vi "Read GObjects.vi"(8 "error in (no error)":errorcluster, 11 "LangData in":refnum<class "VI Data.lvclass">) -> (0 "error out":errorcluster, 2 "GObjects":refnum<class "GObject.lvclass">[](array[class]), 3 "LangData out":refnum<class "VI Data.lvclass">)   [LabVIEW 2013, in "SET Project Data.lvlib" / "VI Data.lvclass"]
uses:
  VI Data.lvclass
  Control Classes/GObject/GObject.lvclass
  VI Data.lvclass/VI Data.ctl
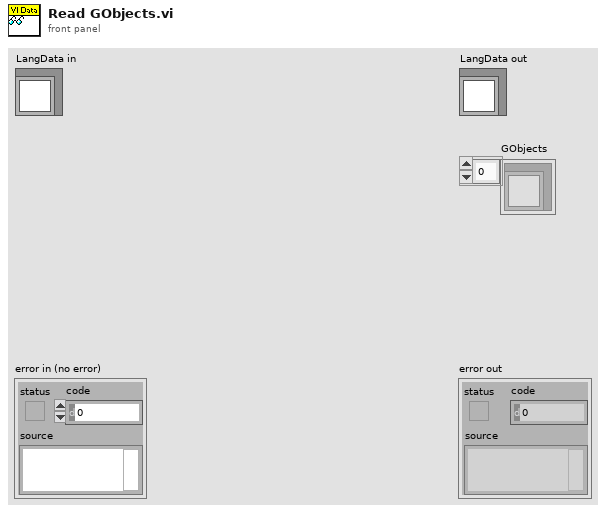
[diagram p1: front panel]
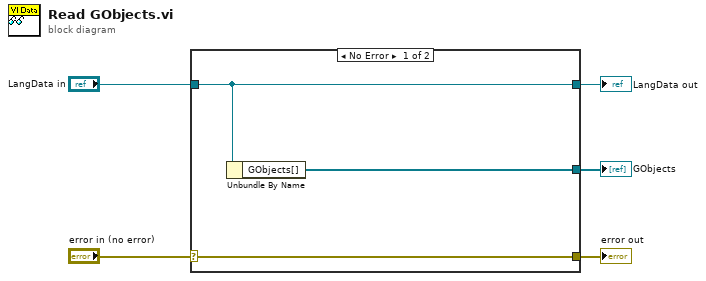
[diagram p0: block diagram]
diagram:
  n1 = case shown="No Error" "error in (no error)" {
    selector: "error in (no error)" -> [w8 w9]
    tunnel: [w8 w9] -> w4
    tunnel: [w7 w10] -> w2
    tunnel: "LangData in" -> [w7 w10]
    tunnel: [w6 _] -> w1
    frame No Error {
      n2 = Unbundle By Name(w7) -> ("GObjects[]"=w6:refnum<class "GObject.lvclass">[])
    }
    frame Error {
    }
  }
  "error out" <- w4
  "LangData out" <- w2
  "GObjects" <- w1
